vi "SWERVE DRIVE.vi"(8 "error in (no error)":errorcluster, 11 "controller in":T6) -> (0 "error out":errorcluster, 3 "controller out":T6)   [LabVIEW 2023]
uses:
  ctrl defs/ctrl controllers.ctl
  ctrl defs/ctrl Logitech Extreme 3D Pro-buttons.ctl
  ctrl defs/ctrl DRIVER MODE.ctl
  ctrl defs/ctrl LimeLight target.ctl
  ctrl defs/ctrl DRIVER target assist.ctl
  ctrl defs/ctrl Logitech Extreme 3D Pro-axis.ctl
  Global odometry.vi
panel:
  out "Driver Assist":T1
  out "Limelight target":T2
  out "coeff/max":dbl=0.13333333333333333
  out "steer max\nVBus":dbl=0.75
  out "DRIVER MODE":T3
  out "BRNG (deg)":dbl format="%.3g"
  out "LOCKED\nand\nCOMMIT":bool
  out "final\nJr to drive":dbl format="%.4g"
  out "target adjustment\nto rotation":dbl format="%.4g"
  in  "rotation coeff":dbl=0.1 format="%.4f"
  out "TARGET ASSIST?":bool
  out "Jr \nfrom\nJoystick":dbl format="%.3g"
  in  "button index\nfor TARGET ASSIST":T4=enum."btn #12"
  in  "button index\nfor DISABLE\nROTATION":T4=enum."btn #3"
  in  "button index\nfor TURTLE":T4=enum."left-side thumb"
  in  "button index\nfor TURBO":T4
  in  "button index\nfor STRAFE\nSTEER = OFF":T4=enum."btn #3"
  in  "Reset\nFILTER":bool
  in  "apply\nFILTER":bool
  in  "sector width (deg)":dbl(ring)=45.0 format="%#_13g" items=["4-sectors"=90.0, "6-sectors"=60.0, "8-sectors"=45.0, "12-sectors"=30.0, "24-sectors"=15.0, ""=0.0]
  out "Buttons":bool[](array[boolean])
  out "POVs":i16[](array[numeric])=[-1]
  out "Axes":dbl[](array[numeric])=[-0.007874015748031496, -0.007874015748031496, 0.0, 0.0]
  in  "select drive controller":T5(ring)=enum."Logitech Extreme 3D Pro"
  in  "notes":string="Joystick 0 - pilot\n\n\"select drive controller\" modifies the X, Y, and twist axis\n\nbutton is momentary STRAFE OFF (usually the driver's thumb)\n\nTURBO and TURTLE added to 0/1  (trigger and thumb)\n\nPOV momentarily modifies rotation center to extreme bumper corners\n\nadded button 11 to activate driver target assist"
  # "NOTE target driver assist controls"
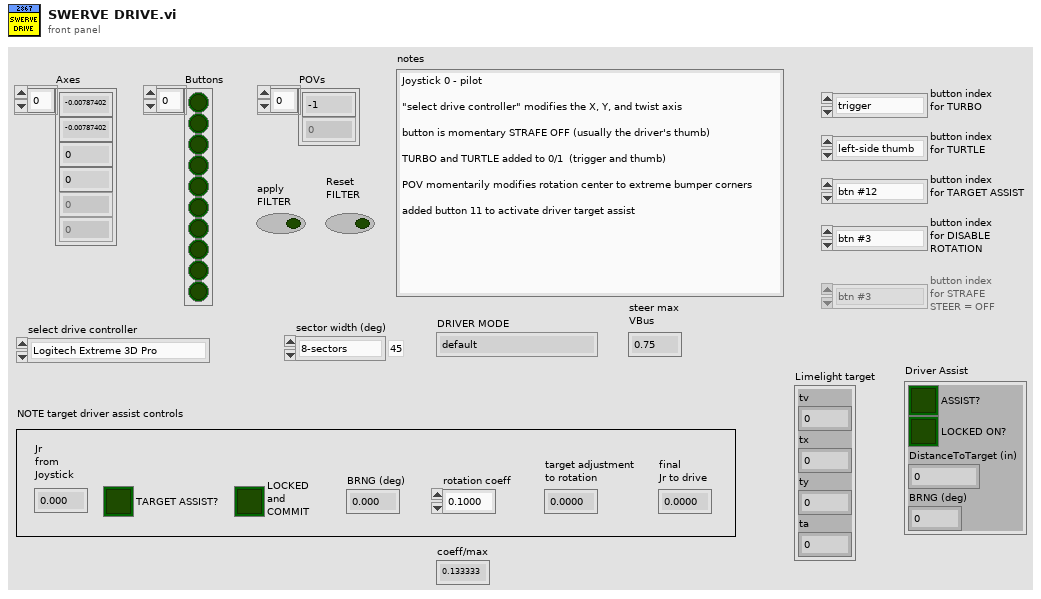
[diagram p1: front panel]
types:
  T1 = typedef "ctrl DRIVER target assist.ctl" = cluster{"ASSIST?":bool, "LOCKED ON?":bool, "DistanceToTarget (in)":dbl, "BRNG (deg)":dbl}
  T2 = typedef "ctrl LimeLight target.ctl" = cluster{"tv":u8, "tx":dbl, "ty":dbl, "ta":dbl}
  T3 = typedef "ctrl DRIVER MODE.ctl" = enum16{"default", "TURTLE", "TURBO"}
  T4 = typedef "ctrl Logitech Extreme 3D Pro-buttons.ctl" = enum16{"trigger", "left-side thumb", "btn #3", "btn #4", "btn #5", "btn #6", "btn #7", "btn #8", "btn #9", "btn #10", "btn #11", "btn #12"}
  T5 = enum16{"Logitech Gamepad", "Mad Katz joystick", "Logitech Extreme 3D Pro"}
  T6 = typedef "ctrl controllers.ctl" = cluster{"Axes":dbl[], "Buttons":bool[], "POVs":i16[]}
  T7 = enum16{"Left X", "Left Y", "Left trigger", "Right trigger", "Right X", "Right Y"}
  T8 = typedef "ctrl Logitech Extreme 3D Pro-axis.ctl" = enum32{"X axis", "Y axis", "Twist", "Throttle"}
  T9 = typedef "ctrl swerve speeds.ctl" = cluster{"NORMAL":cluster{"DRIVE":dbl, "STEER":dbl}, "TURTLE":cluster{"DRIVE":dbl, "STEER":dbl}, "TURBO":cluster{"DRIVE":dbl, "STEER":dbl}}
  T10 = typedef "ctrl driver input.ctl" = cluster{"Jx":dbl, "Jy":dbl, "Jr ":dbl, "R":dbl, "theta (deg)":dbl, "theta (rad)":dbl, "PARK":bool}
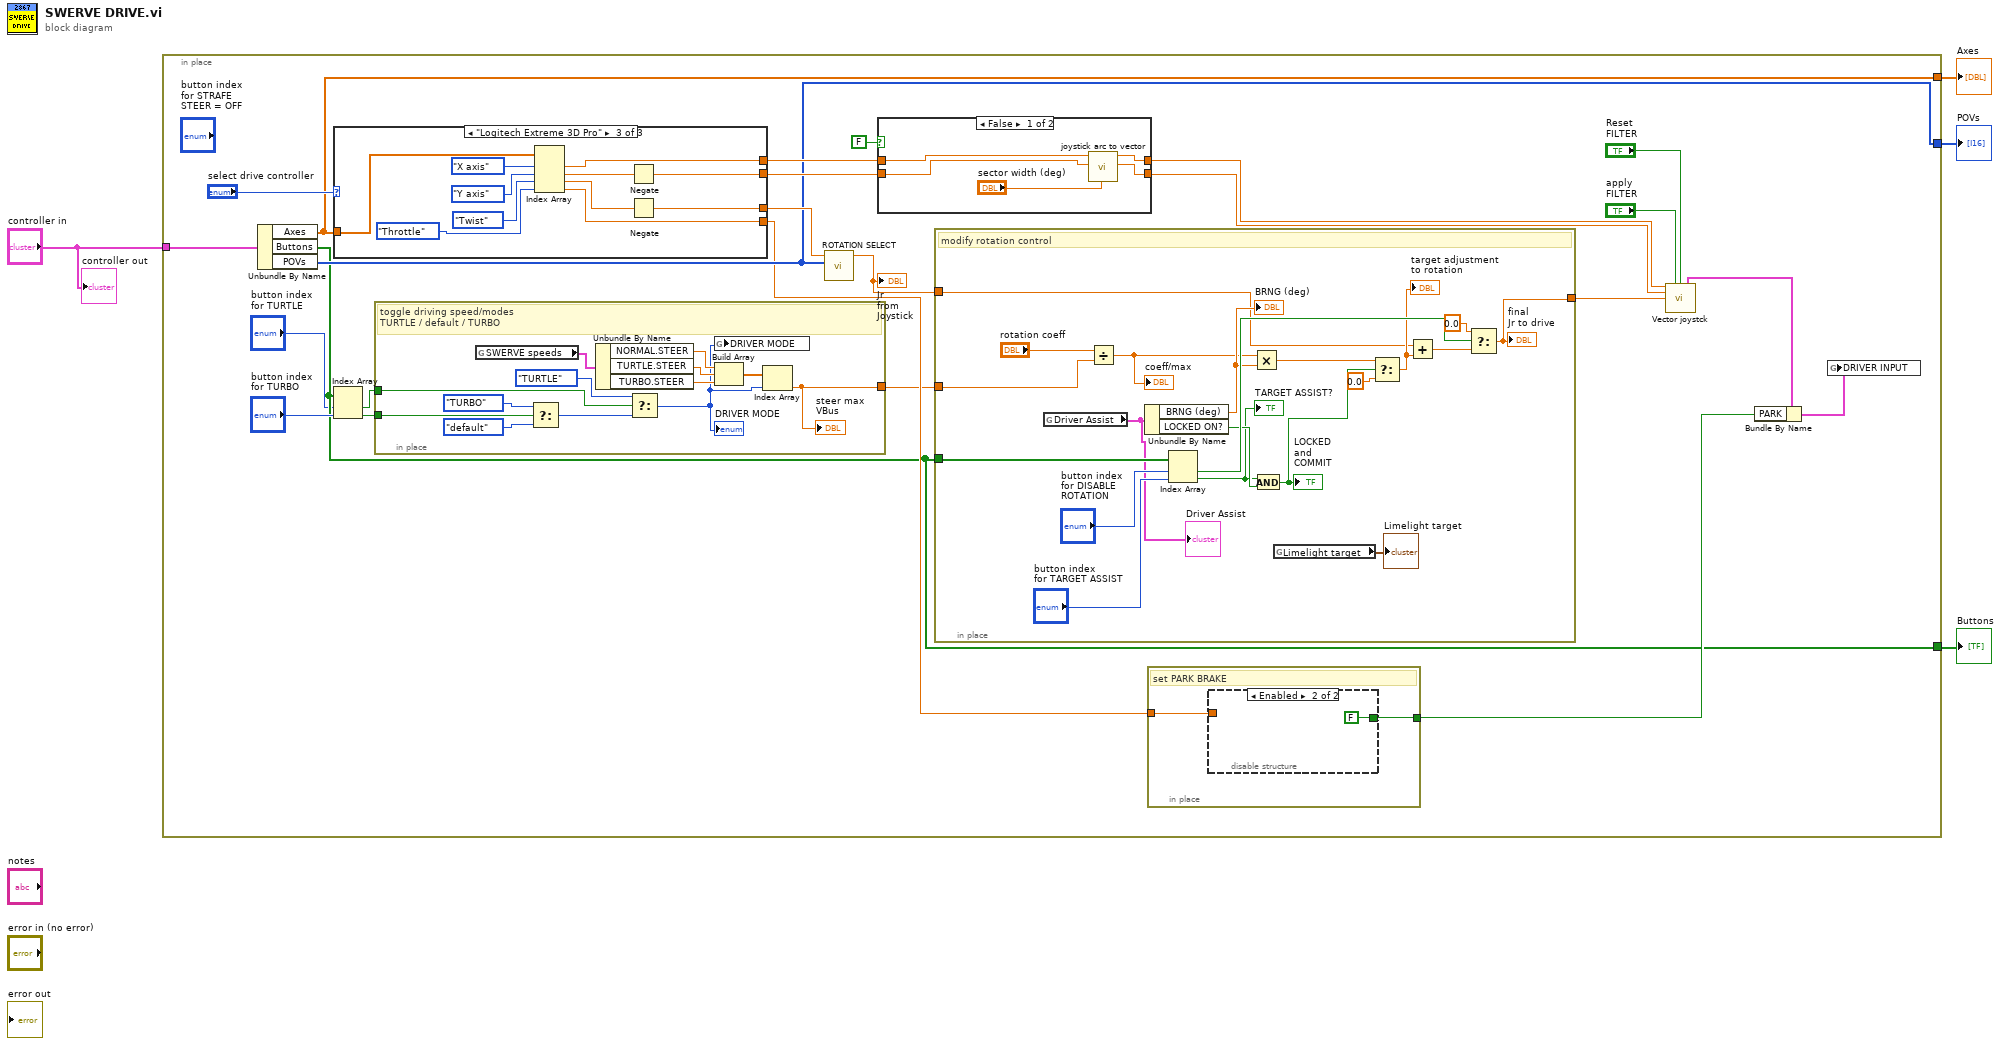
[diagram p0: block diagram]
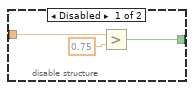
[diagram p2: hidden frame]
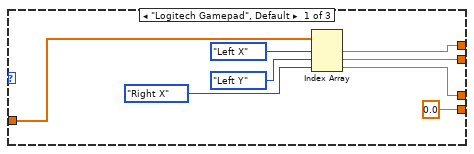
[diagram p4: hidden frame]
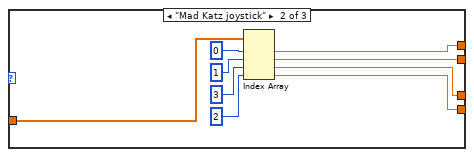
[diagram p5: hidden frame]
diagram:
  n1 = in-place {
    in-place-border: "controller in" -> [w25]
    in-place-border: [w16] -> w3
    in-place-border: [w9] -> w2
    in-place-border: [w15] -> w1
    n2 = Unbundle By Name(w25) -> ("Axes"=w16:dbl[], "Buttons"=w9:bool[], "POVs"=w15:i16[])
    n3 = case shown="\"Logitech Extreme 3D Pro\"" "select drive controller" {
      tunnel: w16 -> [w79 w91 w102]
      tunnel: [w82 w90 w101] -> w22
      tunnel: [w81 w89 w97] -> w21
      tunnel: [w80 w88 w98] -> w26
      tunnel: [0.0 ("upper limit") w83 w96] -> w14
      frame "Logitech Gamepad", Default {
        n4 = Index Array(array=w79, index #1=T7."Left X", index #2=T7."Left Y", index #3=T7."Right X") -> (element #1=w82:dbl, element #2=w81:dbl, element #3=w80:dbl)
      }
      frame "Mad Katz joystick" {
        n5 = Index Array(array=w91, index #1=0 ("index"), index #2=1 ("index"), index #3=3 ("index"), index #4=2 ("index")) -> (element #1=w90:dbl, element #2=w89:dbl, element #3=w88:dbl, element #4=w83:dbl)
      }
      frame "Logitech Extreme 3D Pro" {
        n6 = Index Array(array=w102, index #1=ctrl_Logitech_Extreme_3D_Pro-axis."X axis" ("Logitech Extreme 3D Pro-axis"), index #2=ctrl_Logitech_Extreme_3D_Pro-axis."Y axis" ("Logitech Extreme 3D Pro-axis"), index #3=ctrl_Logitech_Extreme_3D_Pro-axis."Twist" ("Logitech Extreme 3D Pro-axis"), index #4=ctrl_Logitech_Extreme_3D_Pro-axis."Throttle" ("Logitech Extreme 3D Pro-axis")) -> (element #1=w101:dbl, element #2=w100:dbl, element #3=w99:dbl, element #4=w96:dbl)
        n7 = Negate(x=w100) -> (-x=w97:dbl)
        n8 = Negate(x=w99) -> (-x=w98:dbl)
      }
    }
    n9 = Index Array(array=w9, index #1="button index\nfor TURTLE", index #2="button index\nfor TURBO") -> (element #1=w7:bool, element #2=w19:bool)
    n10 = in-place {
      in-place-border: w7 -> [w67]
      in-place-border: w19 -> [w64]
      in-place-border: [w55] -> w6
      # "toggle driving speed/modes\nTURTLE / default / TURBO"
      n11 = global read "Global odometry.vi" "SWERVE speeds"() -> (w57:T9)
      n12 = Select(t=ctrl_DRIVER_MODE."TURBO" ("DRIVER MODE"), s=w64, f=ctrl_DRIVER_MODE."default" ("DRIVER MODE")) -> (s? t:f=w65:T3)
      n13 = Unbundle By Name(w57) -> ("NORMAL.STEER"=w58:dbl, "TURTLE.STEER"=w59:dbl, "TURBO.STEER"=w60:dbl)
      n14 = Select(t=ctrl_DRIVER_MODE."TURTLE" ("DRIVER MODE"), s=w67, f=w65) -> (s? t:f=w56:T3)
      "DRIVER MODE" <- w56
      n15 = global write "Global odometry.vi" "DRIVER MODE"(w56) -> ()
      n16 = Build Array(w58, w59, w60) -> (w61:dbl[])
      n17 = Index Array(array=w61, index=w56) -> (element=w55:dbl)
      "steer max\nVBus" <- w55
    }
    n18 = call "ROTATION SELECT.vi"("POVs in"=w15, "TWIST in"=w26) -> ("Jr"=w11:dbl)  [unwired: 9 in]
    "Jr \nfrom\nJoystick" <- w11
    n19 = case shown="False" FALSE {
      tunnel: [w72 w74] -> w24
      tunnel: [w71 w73] -> w23
      tunnel: w22 -> [w70 w74]
      tunnel: w21 -> [w69 w73]
      frame False {
        n20 = call "joystick arc to vector.vi"("Jx"=w70, "Jy"=w69, "sector width (deg)"="sector width (deg)") -> ("Jx"=w72:dbl, "Jy"=w71:dbl)  [unwired: 13 in, 2 out]
      }
      frame True {
      }
    }
    n21 = in-place {
      in-place-border: [w48] -> w12
      in-place-border: w11 -> [w34]
      in-place-border: w9 -> [w45]
      in-place-border: w6 -> [w31]
      # "modify rotation control"
      n22 = global read "Global odometry.vi" "Driver Assist"() -> (w30:T1)
      "Driver Assist" <- w30
      n23 = Divide(x="rotation coeff", y=w31) -> (x/y=w33:dbl)
      "coeff/max" <- w33
      n24 = Unbundle By Name(w30) -> ("BRNG (deg)"=w37:dbl, "LOCKED ON?"=w42:bool)
      "BRNG (deg)" <- w37
      n25 = Index Array(array=w45, index #1="button index\nfor DISABLE\nROTATION", index #2="button index\nfor TARGET ASSIST") -> (element #1=w44:bool, element #2=w41:bool)
      "TARGET ASSIST?" <- w41
      n26 = Multiply(x=w33, y=w37) -> (x*y=w39:dbl)
      n27 = And(x=w41, y=w42) -> (x .and. y?=w38:bool)
      "LOCKED\nand\nCOMMIT" <- w38
      n28 = global read "Global odometry.vi" "Limelight target"() -> (→"Limelight target":T2)
      n29 = Select(t=w39, s=w38, f=0.0) -> (s? t:f=w40:dbl)
      "target adjustment\nto rotation" <- w40
      n30 = Add(x=w34, y=w40) -> (x+y=w35:dbl)
      n31 = Select(t=0.0, s=w44, f=w35) -> (s? t:f=w48:dbl)
      "final\nJr to drive" <- w48
    }
    n32 = in-place {
      in-place-border: w14 -> [w50]
      in-place-border: [w49] -> w13
      # "set PARK BRAKE"
      n33 = disable-structure shown="Enabled" {
        disable-tunnel: w50 -> [w53 _]
        disable-tunnel: [w51 FALSE] -> w49
        frame Disabled {
          n34 = Greater?(x=w53, y=0.75) -> (0:w51:bool)
        }
        frame Enabled {
        }
      }
    }
    n35 = call "Vector joystck.vi"("Jx input"=w24, "apply\nFILTER"="apply\nFILTER", "Reset\nFILTER"="Reset\nFILTER", "Jy input"=w23, "Jr input"=w12) -> ("output cluster"=w5:T10)  [unwired: 3 in, 7 out]
    n36 = Bundle By Name(cluster=w5, "PARK"=w13) -> (w27:T10)
    n37 = global write "Global odometry.vi" "DRIVER INPUT"(w27) -> ()
  }
  "Axes" <- w3
  "Buttons" <- w2
  "POVs" <- w1
  "controller out" <- "controller in"
